vi "Beat.vi"(7 "Name (\"\" to Use UUID)":string="Beat") -> ()   [LabVIEW 2025]
doc: "Compact code template used to create a CSM module with a user interface. This template includes a user Event Structure for responding to user actions. The functionality of this template is identical to the CSM User Interface(UI) Module Template VI.\n\n\n> [!NOTE] <b>CSM Naming Rules</b>\n>\n> - CSM module name must be unique. Otherwise, CSM enters a `Critical Error` state.\n> - If the input module name is an empty string (\"\"), the system uses a UUID as the module name. Such a module is marked as standalone mode and does not appear in the module list.\n> - Worker Mode Rule: If the input module name ends with `#`, a worker mode node will be instantiated. Multiple worker mode nodes can form a worker mode module.\n> - Chain of Responsibility Mode Rule: If the input module name ends with `$` followed by a number, a chain of responsibility mode node will be instantiated. Multiple chain of responsibility mode nodes can form a chain of responsibility mode module.\n> - System-Level Module Rule: If the input module name starts with `.`, the module is a system-level module. Under default settings, such modules are not listed by the CSM - List Modules VI and are suitable for instantiating modules that run in the background.\n> - Submodule Rule: `.` is also allowed in a module name to separate the module name into multiple parts. CSM does not have strict rules for submodules. The `.` in the module name only marks the logical relationship between different modules. From an execution perspective, they are considered independent modules. The only difference is that you can obtain a list of logical submodules via the CSM - List Submodules VI.\n\n\n-- <b>Controls</b> --\n- <b>Name (\"\" to use UUID)</b>: CSM module name. Refer to <b>CSM Naming Rules</b> for module naming rules."
uses:
  <userlib>/_NEVSTOP/Communicable State Machine(CSM)/AdvanceAPI/CSM - Revert Arguments-Safe String.vi
  <userlib>/_NEVSTOP/Communicable State Machine(CSM)/_Shared/Trim Single-line Text.vi
  <userlib>/_NEVSTOP/Communicable State Machine(CSM)/AdvanceAPI/CSM - Break Down Multiple States String.vi
  <userlib>/_NEVSTOP/Communicable State Machine(CSM)/AdvanceAPI/CSM - Compact Multiple States.vi
  <userlib>/_NEVSTOP/Communicable State Machine(CSM)/AdvanceAPI/CSM - Make String Arguments Safe.vi
  <userlib>/_NEVSTOP/Communicable State Machine(CSM)/AdvanceAPI/CSM - Keywords.vi
  <userlib>/_NEVSTOP/Communicable State Machine(CSM)/Communicable State Machine.lvlib
panel:
  out "Next Beat":dbl
  out "Current Time":u32
  out "x >= y?":bool
  out "N":i32
  out "BeatInterval Indicator":dbl
  out "T0 indicator":dbl
  out "BeatActive":bool
  out "To exit":bool
  out "State History":string
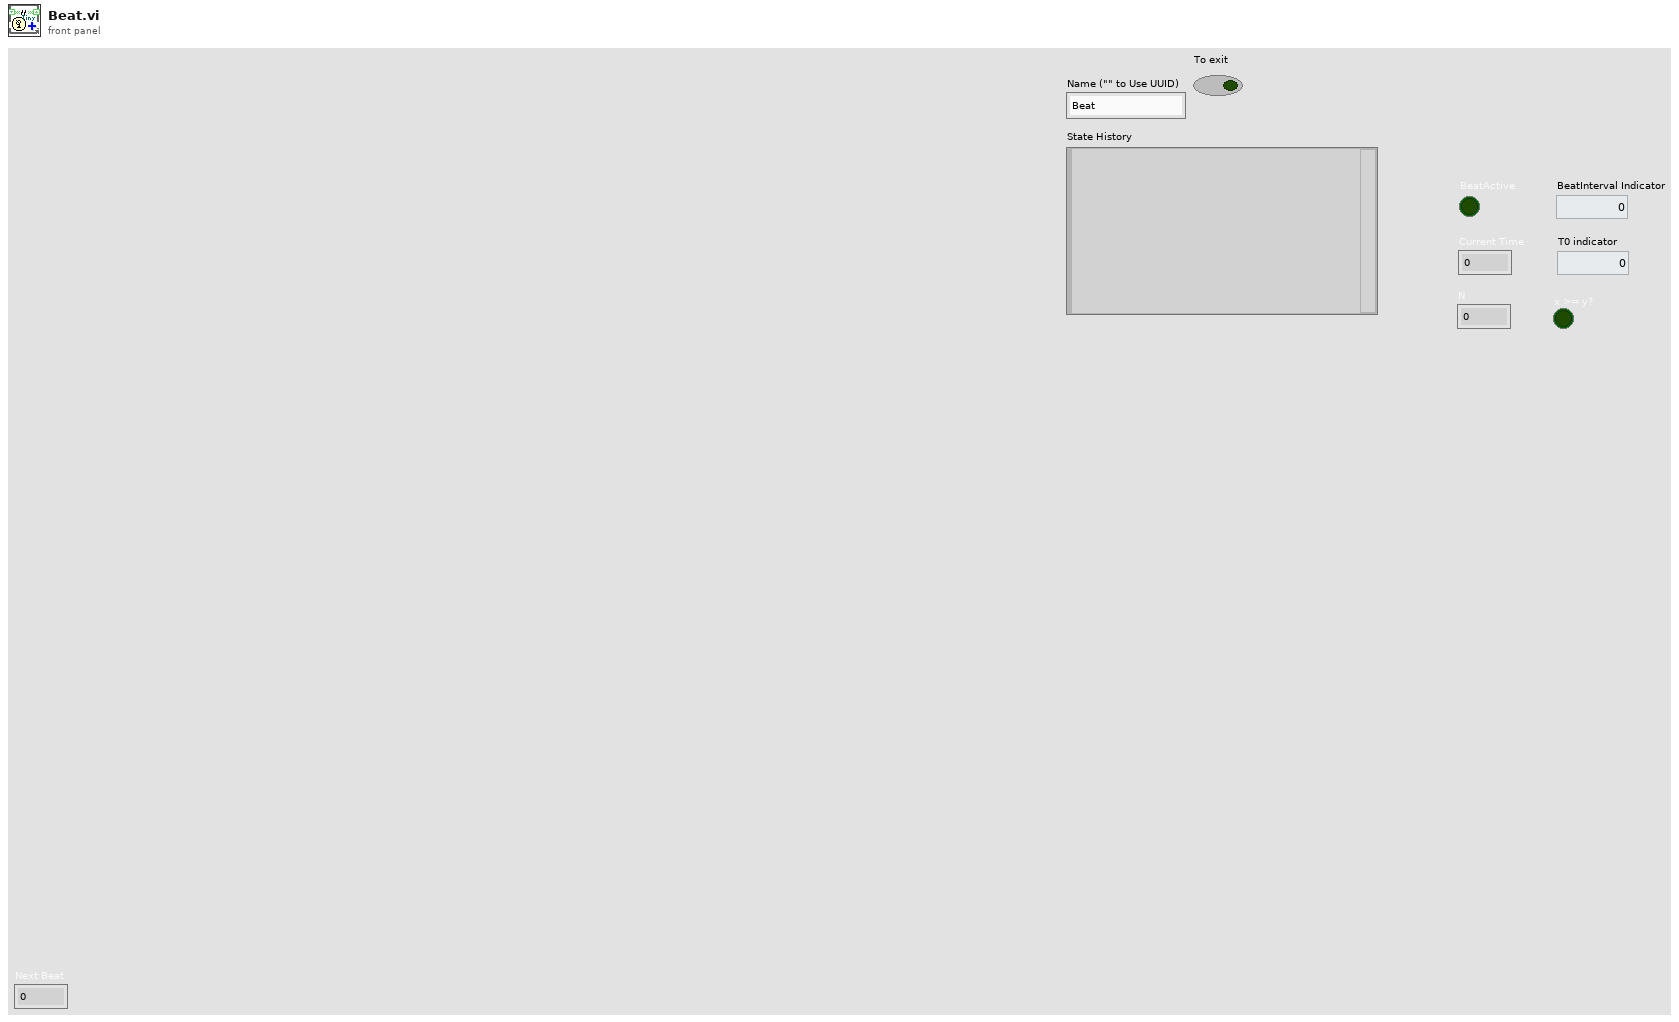
[diagram p1: front panel]
types:
  T1 = enum32{"Invalid", "Standard", "Closed", "Hidden", "Minimized", "Maximized"}
  T2 = enum32{"invalid app kind", "Development System", "Run Time System", "Student Edition", "Embedded LabVIEW", "Evaluation", "Custom"}
  T3 = typedef "Communicable State Machine.lvlib/_CSM_Response Source Message.ctl" = cluster{"‘State":string, "’Arguments":string, "’Error":errorcluster}
  T4 = cluster{"Current VI Reference":refnum<vi>, "Close Panel on Exit?":bool}
  T5 = cluster{"Core":cluster{"Current VI Reference":refnum<vi>, "Close Panel on Exit?":bool}, "T0":u32, "BeatInterval":i32, "BeatActive":bool}
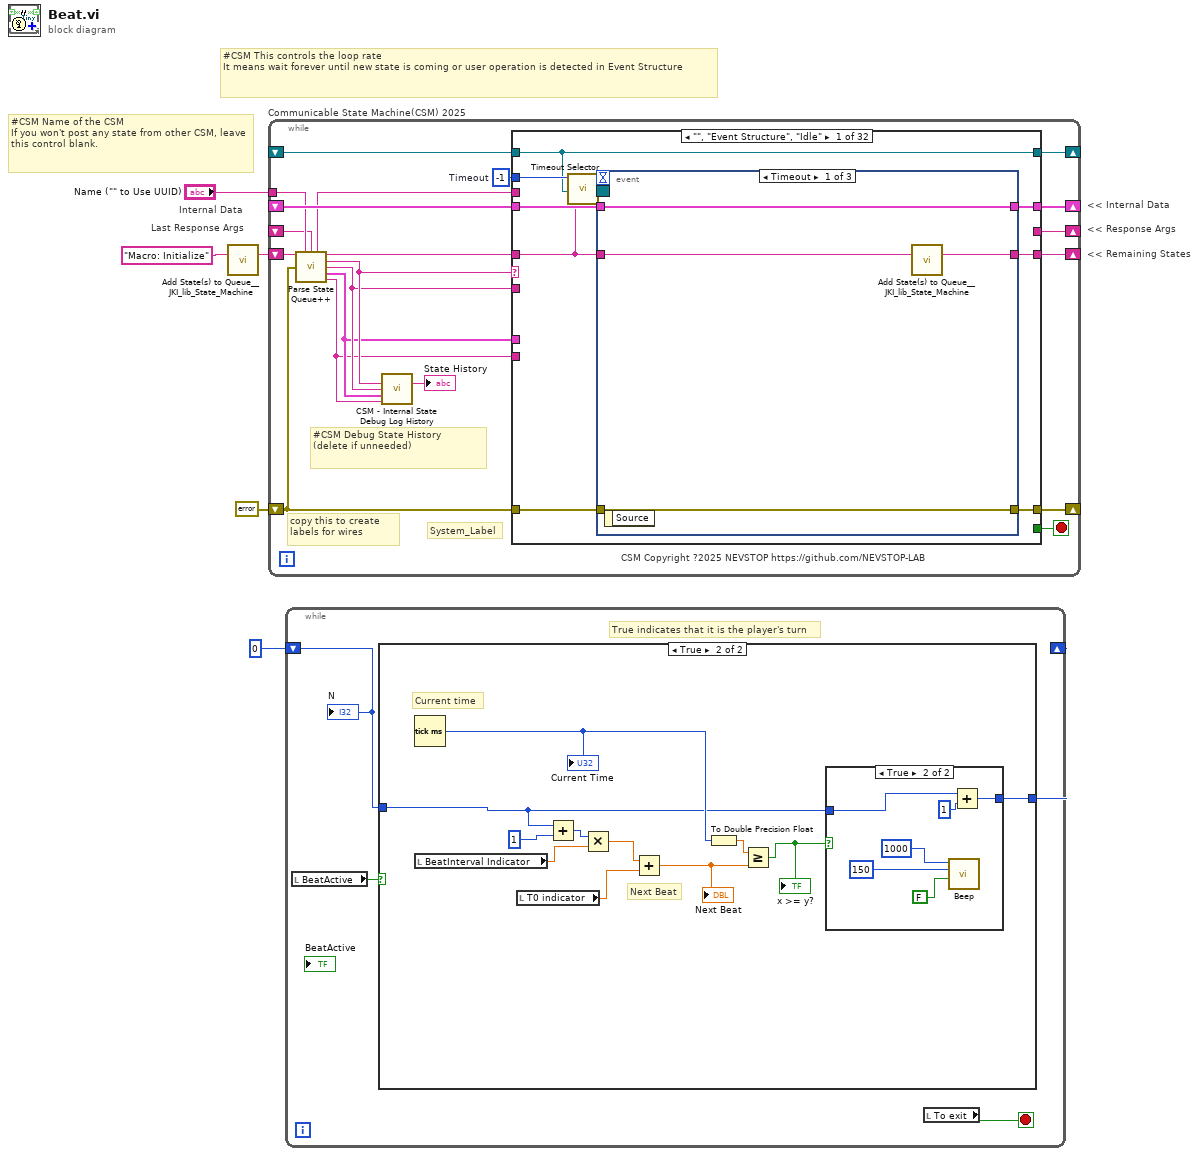
[diagram p0: block diagram]
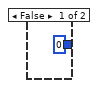
[diagram p2: hidden frame]
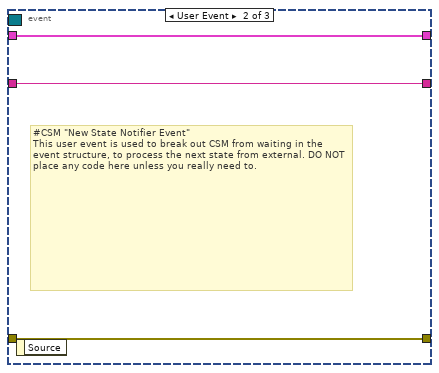
[diagram p4: hidden frame]
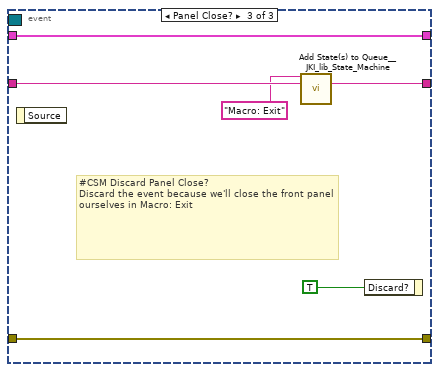
[diagram p5: hidden frame]
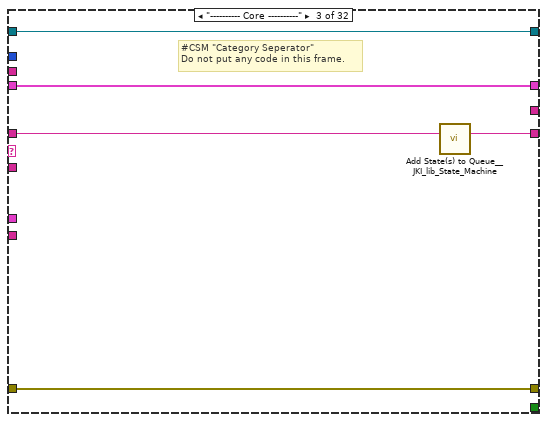
[diagram p7: hidden frame]
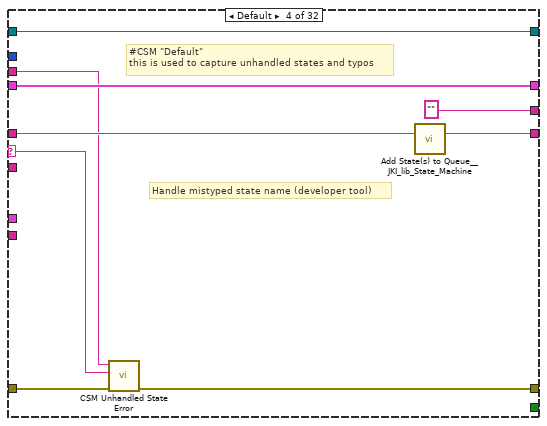
[diagram p8: hidden frame]
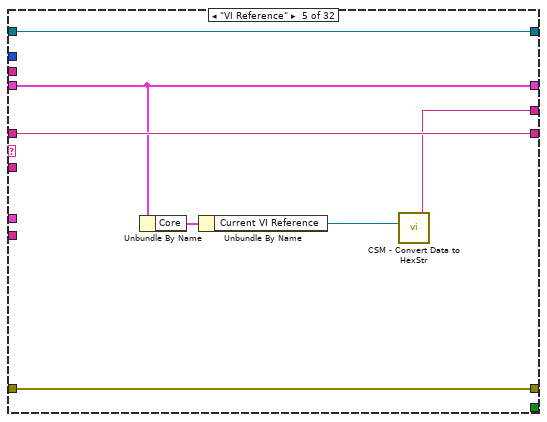
[diagram p9: hidden frame]
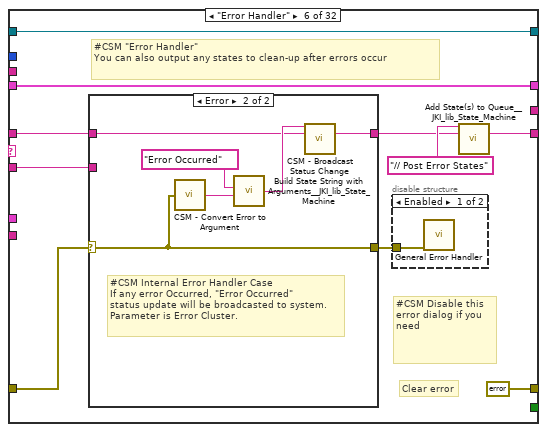
[diagram p10: hidden frame]
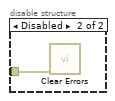
[diagram p11: hidden frame]
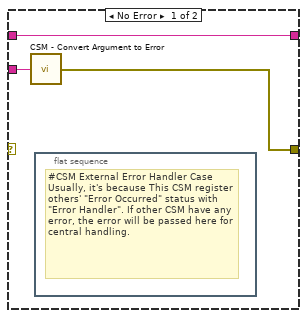
[diagram p12: hidden frame]
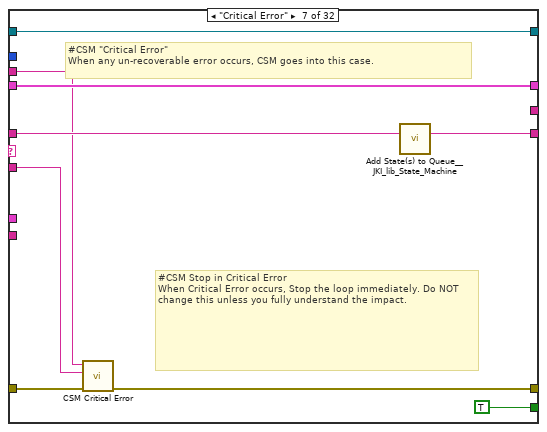
[diagram p13: hidden frame]
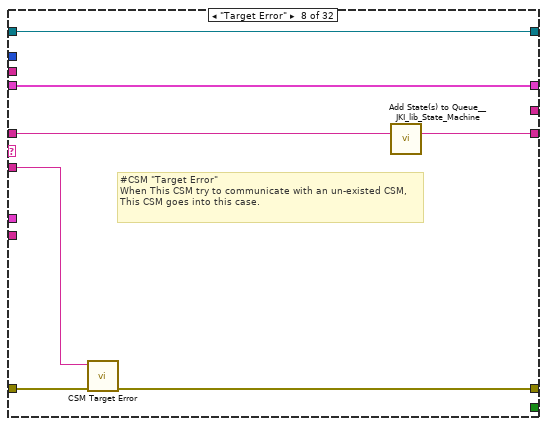
[diagram p14: hidden frame]
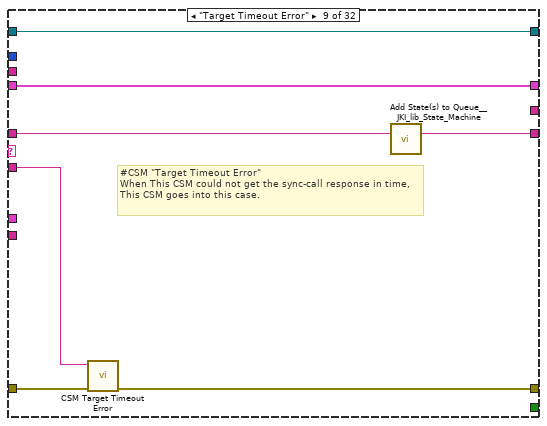
[diagram p15: hidden frame]
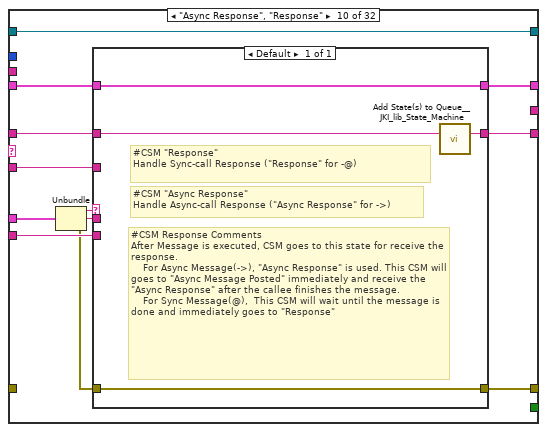
[diagram p16: hidden frame]
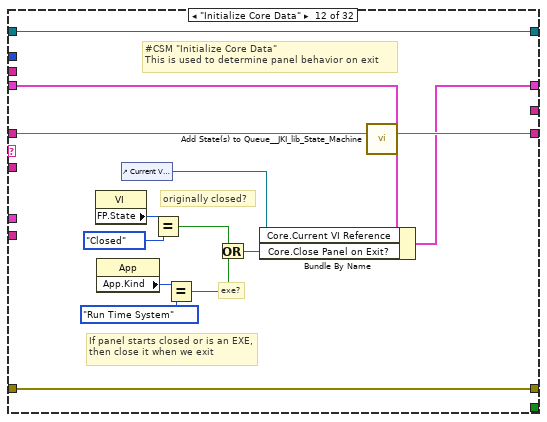
[diagram p18: hidden frame]
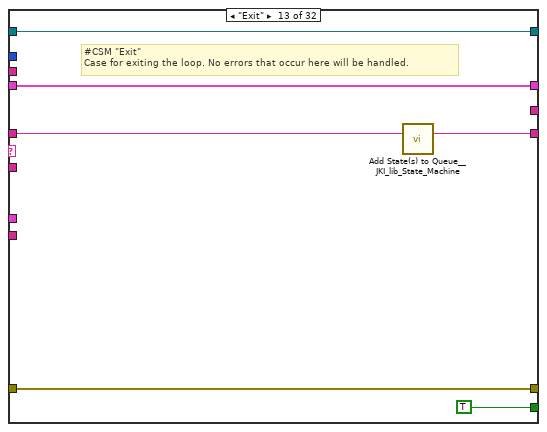
[diagram p19: hidden frame]
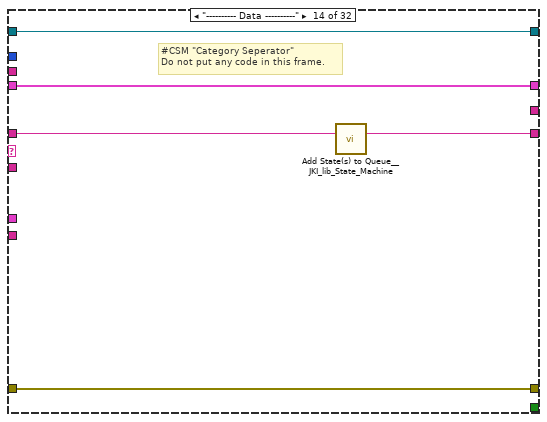
[diagram p20: hidden frame]
diagram:
  # "Last Response Args"
  # "Internal Data"
  # "#CSM Name of the CSM\nIf you won't post any state from other CSM, leave this control blank."
  # "#CSM This controls the loop rate\nIt means wait forever until new state is coming or user operation is detected in Event Structure"
  # "<< Internal Data"
  # "<< Response Args"
  # "<< Remaining States"
  n1 = call <vilib>:"Add State(s) to Queue__JKI_lib_State_Machine.vi"("State(s) in (\"\")"="Macro: Initialize" ("Init State(\"Macro: Initialize\")")) -> ("States Out"=w5:string)  [unwired: 14 in]
  n2 = while "Communicable State Machine(CSM) 2025" {
    shift-right: [w20] -> _
    shift-left: _ -> [w19]
    shift-right: [w23] -> _
    shift-left: errorcluster {"status"=FALSE, "code"=0, "source"=""} ("error out") -> [w17]
    shift-right: [w22] -> _
    shift-left: w5 -> [w24]
    tunnel: "Name (\"\" to Use UUID)" -> [w13]
    shift-right: [w16] -> _
    shift-left: _ -> [w7]
    shift-right: [w15] -> _
    shift-left: _ -> [w14]
    stop <- w21 stop-if-true
    w18 = -1  # Timeout
    # "#CSM Debug State History\n(delete if unneeded)"
    # "copy this to create labels for wires"
    # "System_Label"
    # "CSM Copyright ?2025 NEVSTOP https://github.com/NEVSTOP-LAB"
    n3 = call <userlib>:"Parse State Queue++.vi"("State Queue"=w24, "Name (\"\" to Use UUID)"=w13, "Response Arguments"=w7, "Previous Error"=w17) -> ("Name Used"=w8:string, "Remaining States"=w25:string, "Current State"=w12:string, "Arguments"=w11:string, "Additional Information"=w10:T3, "Source CSM"=w9:string)  [unwired: 6 in]
    n4 = call <userlib>:"CSM - Internal State Debug Log History.vi"("State"=w12, "Arguments (\"\")"=w11, ">> Response Source Message >>"=w10, "Source (\"\")"=w9) -> ("Debug Log"=→"State History":string)  [unwired: 11 in]
    n5 = case shown="\"\", \"Event Structure\", \"Idle\"" w12 {
      selector: w12 -> [_ _ _ w59 _ _ _ _ _ _ _ _ _ _ _ _ _ _ _ _ _ _ _ _ _ _ _ _ _ _ _ _]
      tunnel: w25 -> [w26 w50 w56 w64 w71 w77 w100 w106 w113 w122 w135 w150 w156 w161 w170 w177 w182 w189 w193 w199 w204 w211 w227 w297 w303 w315 w318 w334 w338 w349 w357 w362]
      tunnel: w11 -> [_ _ _ _ _ w76 w95 w105 w112 w121 _ _ _ _ _ _ _ _ _ _ _ w206 w221 _ _ _ _ w328 _ _ _ _]
      tunnel: w19 -> [w33 w49 w53 w62 w70 w81 w101 w108 w115 w124 w134 w143 w154 w158 _ w172 w179 w188 w192 w196 w202 w209 w223 w294 w300 w312 w317 w331 w343 w346 w353 w359]
      tunnel: [w32 w51 w54 w57 w72 errorcluster {"status"=FALSE, "code"=0, "source"=""} ("error out") w96 w103 w110 w127 w136 w147 w153 w159 w167 w173 w180 w183 w191 w197 w201 w207 w224 w295 w301 w313 w319 w335 w344 w347 w355 w360] -> w23
      tunnel: w17 -> [w31 w51 w54 w65 w72 w78 w102 w104 w111 _ w136 w147 w153 w159 w167 w174 w180 _ w194 w197 w201 w208 w225 w295 w301 w313 w319 w335 w344 w347 w355 w360]
      tunnel: [w34 w50 w55 w63 w71 w73 w99 w109 w116 w123 w135 w149 w155 w160 w169 w176 w181 w189 w193 w198 w203 w210 w226 w296 w302 w314 w318 w334 w337 w348 w356 w361] -> w22
      tunnel: [_ _ _ _ _ _ TRUE _ _ _ _ _ TRUE _ _ _ _ _ _ _ _ _ _ _ _ _ _ _ _ _ _ _] -> w21
      tunnel: [w30 w49 w53 w62 w70 w81 w101 w108 w115 w125 w134 w148 w154 w158 w168 w172 w179 w188 w192 w196 w202 w209 w223 w294 w300 w312 w317 w330 w343 w346 w350 w359] -> w20
      tunnel: w18 -> [w29 _ _ _ _ _ _ _ _ _ _ _ _ _ _ _ _ _ _ _ _ _ _ _ _ _ _ _ _ _ _ _]
      tunnel: w9 -> [_ _ _ _ _ _ _ _ _ w119 _ _ _ _ _ _ _ _ _ _ _ _ _ _ _ _ _ _ _ _ _ _]
      tunnel: w10 -> [_ _ _ _ _ _ _ _ _ w126 _ _ _ _ _ _ _ _ _ _ _ _ _ _ _ _ _ _ _ _ _ _]
      tunnel: [_ _ _ "" w66 _ _ _ _ _ _ _ _ _ _ _ _ _ _ _ _ _ _ _ _ _ _ "API1 Response" "API2 Response" _ _ _] -> w16
      tunnel: [w28 w48 w52 w60 w69 w80 w97 w107 w114 w128 w133 w137 w151 w157 w165 w171 w178 w187 w190 w195 w200 w205 w220 w293 w298 w305 w316 w333 w342 w345 w354 w358] -> w15
      tunnel: w14 -> [w28 w48 w52 w60 w69 w80 w97 w107 w114 w128 w133 w137 w151 w157 w165 w171 w178 _ w190 w195 w200 w205 w220 w293 w298 w305 w316 w333 w342 w345 w354 w358]
      tunnel: w8 -> [_ _ _ w58 _ _ w94 _ _ _ _ _ _ _ _ _ _ w186 _ _ _ _ _ _ _ _ _ _ _ _ _ _]
      frame "", "Event Structure", "Idle" {
        n6 = call <userlib>:"Timeout Selector.vi"("Remaining States"=w26, "Timeout Expected"=w29) -> ("Timeout"=w27:i32)  [unwired: 5 in]
        n7 = event shown="[0] Timeout" {
          selector: w28 -> [_ _ _]
          dyn-events: _ -> [_ _ _]
          timeout: w27 -> [_ _ _]
          tunnel: w26 -> [w38 w40 w47]
          tunnel: [w37 w40 w46] -> w34
          tunnel: w33 -> [w35 w41 w44]
          tunnel: [w36 w39 w45] -> w32
          tunnel: w31 -> [w36 w39 w45]
          tunnel: [w35 w41 w44] -> w30
          event Timeout {
            n8 = event-data() -> ()  [unwired: 1 in, 1 out]
            n9 = call <vilib>:"Add State(s) to Queue__JKI_lib_State_Machine.vi"("State(s) in (\"\")"=w38) -> ("States Out"=w37:string)  [unwired: 14 in]
          }
          event User Event {
            # "#CSM \"New State Notifier Event\"\nThis user event is used to break out CSM from waiting in the event structure, to process the next state from external. DO NOT place any code here unless you really need to."
            n10 = event-data() -> ()  [unwired: 1 in, 1 out]
          }
          event Panel Close? {
            # "#CSM Discard Panel Close?\nDiscard the event because we'll close the front panel ourselves in Macro: Exit"
            n11 = event-data() -> ()  [unwired: 1 in, 1 out]
            n12 = call <vilib>:"Add State(s) to Queue__JKI_lib_State_Machine.vi"("State(s) in Front (\"\")"="Macro: Exit", "State(s) in (\"\")"=w47) -> ("States Out"=w46:string)  [unwired: 13 in]
            n13 = event-data("Discard?"=TRUE) -> ()  [unwired: 1 in, 1 out]
          }
        }
      }
      frame "CSM Documentation" {
        # "#CSM README FIRST\n\nCommunicable State Machine(CSM) is a LabVIEW application framework that builds upon JKI State Machine(JKISM). It follows the pattern of JKISM and extends the keywords to describe message communication between modules, including concepts such as Sync-Message, Async-Message, Subscription/Unsubscription of status - essential elements for creating reusable code modules. For more information, please visit the CSM wiki: https://nevstop-lab.github.io/CSM-Wiki/\n\nFor instructions on JKI State Machine, visit: http://jki.net/state-machine/\nFor information about CSM, visit: https://github.com/NEVSTOP-LAB"
        # "#CSM \"Documentation\"\nCase for holding CSM Documenation"
      }
      frame "---------- Core ----------" {
        # "#CSM \"Category Seperator\"\nDo not put any code in this frame."
        n14 = call <vilib>:"Add State(s) to Queue__JKI_lib_State_Machine.vi"("State(s) in (\"\")"=w56) -> ("States Out"=w55:string)  [unwired: 14 in]
      }
      frame Default {
        # "#CSM \"Default\"\nthis is used to capture unhandled states and typos"
        # "Handle mistyped state name (developer tool)"
        n15 = call <userlib>:"CSM Unhandled State Error.vi"("error in (no error)"=w65, "Undefined State"=w59, "CSM Name"=w58) -> ("error out"=w57:errorcluster)  [unwired: 8 in]
        n16 = call <vilib>:"Add State(s) to Queue__JKI_lib_State_Machine.vi"("State(s) in (\"\")"=w64) -> ("States Out"=w63:string)  [unwired: 14 in]
      }
      frame "VI Reference" {
        n17 = Unbundle By Name(w70) -> ("Core"=w68:T4)
        n18 = Unbundle By Name(w68) -> ("Current VI Reference"=w67:refnum<vi>)
        n19 = call <userlib>:"CSM - Convert Data to HexStr.vi"("Variant"=w67) -> ("HEX String (0-9,A-F)"=w66:string)  [unwired: 8 in]
      }
      frame "Error Handler" {
        # "#CSM Disable this error dialog if you need"
        # "#CSM \"Error Handler\"\nYou can also output any states to clean-up after errors occur"
        # "Clear error"
        n20 = case shown="Error" w78 {
          selector: w78 -> [_ w88]
          tunnel: [w87 w90] -> w74
          tunnel: w77 -> [w87 w89]
          tunnel: w76 -> [w86 _]
          tunnel: [w85 w88] -> w79
          frame No Error {
            n21 = call <userlib>:"CSM - Convert Argument to Error.vi"("Argument"=w86) -> ("Error"=w85:errorcluster)  [unwired: 4 in]
            n22 = flat-sequence {
              frame #0 {
                # "#CSM External Error Handler Case\nUsually, it's because This CSM register others' \"Error Occurred\" status with \"Error Handler\". If other CSM have any error, the error will be passed here for central handling."
              }
            }
          }
          frame Error {
            # "#CSM Internal Error Handler Case \nIf any error Occurred, \"Error Occurred\" \nstatus update will be broadcasted to system.\nParameter is Error Cluster."
            n23 = call <userlib>:"CSM - Convert Error to Argument.vi"("Error"=w88) -> ("Argument"=w92:string)  [unwired: 4 in]
            n24 = call <vilib>:"Build State String with Arguments__JKI_lib_State_Machine.vi"("Arguments (\"\")"=w92, "State"="Error Occurred" ("Status with Arguments")) -> ("State with Arguments"=w91:string)  [unwired: 4 in]
            n25 = call <userlib>:"CSM - Broadcast Status Change.vi"("Status With Arguments"=w91, "State Queue"=w89) -> ("Remaining States"=w90:string)  [unwired: 13 in]
          }
        }
        n26 = disable-structure shown="Enabled" {
          disable-tunnel: w79 -> [w83 w84]
          frame Enabled {
            n27 = call <vilib>:"General Error Handler.vi"("error in (no error)"=w83) -> ()  [unwired: 10 in, 5 out]
          }
          frame Disabled {
            n28 = call <vilib>:"Clear Errors.vi"("error in (no error)"=w84) -> ()  [unwired: 5 in, 2 out]
          }
        }
        n29 = call <vilib>:"Add State(s) to Queue__JKI_lib_State_Machine.vi"("State(s) in Front (\"\")"="// Post Error States", "State(s) in (\"\")"=w74) -> ("States Out"=w73:string)  [unwired: 13 in]
      }
      frame "Critical Error" {
        # "#CSM Stop in Critical Error\nWhen Critical Error occurs, Stop the loop immediately. Do NOT change this unless you fully understand the impact."
        # "#CSM \"Critical Error\"\nWhen any un-recoverable error occurs, CSM goes into this case."
        n30 = call <userlib>:"CSM Critical Error.vi"("error in (no error)"=w102, "Arugments (As Reason)"=w95, "CSM Name"=w94) -> ("error out"=w96:errorcluster)  [unwired: 8 in]
        n31 = call <vilib>:"Add State(s) to Queue__JKI_lib_State_Machine.vi"("State(s) in (\"\")"=w100) -> ("States Out"=w99:string)  [unwired: 14 in]
      }
      frame "Target Error" {
        # "#CSM \"Target Error\"\nWhen This CSM try to communicate with an un-existed CSM, This CSM goes into this case."
        n32 = call <userlib>:"CSM Target Error.vi"("error in (no error)"=w104, "Arguments (As CSM Name)"=w105) -> ("error out"=w103:errorcluster)  [unwired: 9 in]
        n33 = call <vilib>:"Add State(s) to Queue__JKI_lib_State_Machine.vi"("State(s) in (\"\")"=w106) -> ("States Out"=w109:string)  [unwired: 14 in]
      }
      frame "Target Timeout Error" {
        # "#CSM \"Target Timeout Error\"\nWhen This CSM could not get the sync-call response in time, This CSM goes into this case."
        n34 = call <userlib>:"CSM Target Timeout Error.vi"("error in (no error)"=w111, "Arguments (As CSM Name)"=w112) -> ("error out"=w110:errorcluster)  [unwired: 9 in]
        n35 = call <vilib>:"Add State(s) to Queue__JKI_lib_State_Machine.vi"("State(s) in (\"\")"=w113) -> ("States Out"=w116:string)  [unwired: 14 in]
      }
      frame "Async Response", "Response" {
        n36 = Unbundle(w126) -> ("‘State"=w120:string, "’Arguments"=w118:string, "’Error"=w117:errorcluster)
        n37 = case shown="Default" w120 {
          tunnel: [w132] -> w127
          tunnel: w117 -> [w132]
          tunnel: [w131] -> w125
          tunnel: w124 -> [w131]
          tunnel: [w129] -> w123
          tunnel: w122 -> [w130]
          tunnel: w121 -> [_]
          tunnel: w119 -> [_]
          tunnel: w118 -> [_]
          frame Default {
            # "#CSM Response Comments\nAfter Message is executed, CSM goes to this state for receive the response.\n    For Async Message(->), \"Async Response\" is used. This CSM will goes to \"Async Message Posted\" immediately and receive the \"Async Response\" after the callee finishes the message.\n    For Sync Message(@),  This CSM will wait until the message is done and immediately goes to \"Response\""
            # "#CSM \"Async Response\"\nHandle Async-call Response (\"Async Response\" for ->)"
            # "#CSM \"Response\"\nHandle Sync-call Response (\"Response\" for -@)"
            n38 = call <vilib>:"Add State(s) to Queue__JKI_lib_State_Machine.vi"("State(s) in (\"\")"=w130) -> ("States Out"=w129:string)  [unwired: 14 in]
          }
        }
      }
      frame "Async Message Posted" {
        # "#CSM \"Async Message Posted\"\nAfter Async Message is posted (-> or ->| ), CSM goes to this state for post-action.\nYou can use Argument - State to tell which Async Message is called."
      }
      frame "Initialize Core Data" {
        # "#CSM \"Initialize Core Data\"\nThis is used to determine panel behavior on exit"
        # "originally closed?"
        # "exe?"
        # "If panel starts closed or is an EXE, then close it when we exit"
        n39 = property class="VI"() -> ("FP.State"=w140:T1)  [unwired: 2 in, 2 out]
        n40 = property class="App"() -> ("App.Kind"=w146:T2)  [unwired: 2 in, 2 out]
        n41 = control-ref of="Current VI Reference"() -> (w141:refnum<vi>)
        n42 = Equal?(x=w140, y=T1."Closed" ("Front Panel Window:State")) -> (x = y?=w138:bool)
        n43 = Equal?(x=w146, y=T2."Run Time System" ("Application:Kind")) -> (x = y?=w144:bool)
        n44 = Or(x=w138, y=w144) -> (x .or. y?=w142:bool)
        n45 = Bundle By Name(cluster=w143, "Core.Current VI Reference"=w141, "Core.Close Panel on Exit?"=w142) -> (w148:T5)
        n46 = call <vilib>:"Add State(s) to Queue__JKI_lib_State_Machine.vi"("State(s) in (\"\")"=w150) -> ("States Out"=w149:string)  [unwired: 14 in]
      }
      frame "Exit" {
        # "#CSM \"Exit\"\nCase for exiting the loop. No errors that occur here will be handled."
        n47 = call <vilib>:"Add State(s) to Queue__JKI_lib_State_Machine.vi"("State(s) in (\"\")"=w156) -> ("States Out"=w155:string)  [unwired: 14 in]
      }
      frame "---------- Data ----------" {
        # "#CSM \"Category Seperator\"\nDo not put any code in this frame."
        n48 = call <vilib>:"Add State(s) to Queue__JKI_lib_State_Machine.vi"("State(s) in (\"\")"=w161) -> ("States Out"=w160:string)  [unwired: 14 in]
      }
      frame "Data: Initialize" {
        w162 = FALSE  # BeatActive
        w163 = 0  # BeatInterval
        w164 = u32 0  # T0
        w166 = T4 {"Current VI Reference"=refnum, "Close Panel on Exit?"=FALSE}  # Core
        # "#CSM do not delete - used by framework"
        # "#CSM Expand Bundle to add new data elements to shift register data."
        # "#CSM Add new data here."
        # "Initialize the shift-register data, here.\n(data names are defined by what you wire into the bundle function)"
        n49 = Bundle("Core"=w166, "T0"=w164, "BeatInterval"=w163, "BeatActive"=w162) -> (w168:T5)  [unwired: 1 in]
        n50 = call <vilib>:"Add State(s) to Queue__JKI_lib_State_Machine.vi"("State(s) in (\"\")"=w170) -> ("States Out"=w169:string)  [unwired: 14 in]
      }
      frame "Data: Cleanup" {
        # "Cleanup any data and references, here.\n(this is called automatically, by the Macro: Exit)"
        n51 = Unbundle By Name(w172) -> ("Core.Current VI Reference"=w175:refnum<vi>)
        n52 = Close Reference(reference=w175, error in (no error)=w174) -> (error out=w173:errorcluster)
        n53 = call <vilib>:"Add State(s) to Queue__JKI_lib_State_Machine.vi"("State(s) in (\"\")"=w177) -> ("States Out"=w176:string)  [unwired: 14 in]
      }
      frame "---------- Events ----------" {
        # "#CSM \"Category Seperator\"\nDo not put any code in this frame."
        n54 = call <vilib>:"Add State(s) to Queue__JKI_lib_State_Machine.vi"("State(s) in (\"\")"=w182) -> ("States Out"=w181:string)  [unwired: 14 in]
      }
      frame "Events: Register" {
        # "#CSM \"Events: Register\"\nRegister user event. New Message Event is registered to break CSM waiting in event structure by default."
        # "#CSM Register New Message Event\nRegister message event to break Waiting in Event structure."
        n55 = call <userlib>:"CSM - Get New State Notifier Event.vi"("Name (\"\" to Use UUID)"=w186) -> ("error out"=w184:errorcluster, "New State Notifier Event"=w185:refnum<user-event>)  [unwired: 9 in]
        n56 = register-events(error in=w184, w185) -> (reference out=w187:refnum<event-registration>, error out=w183:errorcluster)  [unwired: 1 in]
      }
      frame "Events: Unregister" {
        # "#CSM \"Events: Unregister\"\nUnregister user event."
        n57 = Unregister For Events(event registration refnum=w190, error in=w194) -> (error out=w191:errorcluster)
      }
      frame "---------- UI ----------" {
        # "#CSM \"Category Seperator\"\nDo not put any code in this frame."
        n58 = call <vilib>:"Add State(s) to Queue__JKI_lib_State_Machine.vi"("State(s) in (\"\")"=w199) -> ("States Out"=w198:string)  [unwired: 14 in]
      }
      frame "UI: Initialize" {
        # "#CSM \"UI: Initialize\"\nInitialize the User Interface, here.\n(this is called automatically, by the Macro: Init)"
        n59 = call <vilib>:"Add State(s) to Queue__JKI_lib_State_Machine.vi"("State(s) in (\"\")"=w204) -> ("States Out"=w203:string)  [unwired: 14 in]
      }
      frame "UI: Cursor Set" {
        # "#CSM \"UI: Cursor Set\"\nSet and Unset Cursor Busy.\n(Usage: \"UI: Cursor Set >> Busy|Idle\")"
        # "Argument"
        n60 = disable-structure shown="Default" {
          disable-tunnel: w208 -> [w214 w219]
          disable-tunnel: [w213 w219] -> w207
          disable-tunnel: w206 -> [w212 _]
          frame condition #0 (active) {
            n61 = case shown="\"Idle\", Default" w212 {
              tunnel: w214 -> [w216 w218]
              tunnel: [w215 w217] -> w213
              frame "Idle", Default {
                n62 = call <vilib>:"Unset Busy.vi"("error in (no error)"=w216) -> ("error out"=w215:errorcluster)  [unwired: 10 in]
              }
              frame "Busy" {
                n63 = call <vilib>:"Set Busy.vi"("error in (no error)"=w218) -> ("error out"=w217:errorcluster)  [unwired: 9 in, 1 out]
              }
            }
          }
          frame condition #1 {
          }
        }
        n64 = call <vilib>:"Add State(s) to Queue__JKI_lib_State_Machine.vi"("State(s) in (\"\")"=w211) -> ("States Out"=w210:string)  [unwired: 14 in]
      }
      frame "UI: Front Panel State" {
        # "#CSM \"UI: Front Panel State\"\nSet Front Panel Open or Closed\n(Usage: \"UI: Front Panel State >> Open|Close\")"
        # "Argument"
        n65 = Unbundle By Name(w223) -> ("Core.Current VI Reference"=w222:refnum<vi>)
        n66 = call <vilib>:"Add State(s) to Queue__JKI_lib_State_Machine.vi"("State(s) in (\"\")"=w227) -> ("States Out"=w226:string)  [unwired: 14 in]
        n67 = case shown="\"Close\", \"Closed\"" w221 {
          tunnel: w225 -> [w233 w248 w259 w272 w285]
          tunnel: [w235 w249 w261 w274 w287] -> w224
          tunnel: w222 -> [w234 w246 w260 w273 w286]
          frame "Open", "Standard", Default {
            w228 = T1."Standard" ("State")
            n68 = property class="VI"(reference=w234, error in=w233) -> (reference out=w231:refnum<vi>, error out=w232:errorcluster, "FP.State"=w230:T1)
            n69 = Not Equal?(x=w230, y=w228) -> (x != y?=w229:bool)
            n70 = case shown="True" w229 {
              tunnel: [w239 w241] -> w235
              tunnel: w232 -> [w238 w241]
              tunnel: w231 -> [w237 _]
              tunnel: w228 -> [w236 _]
              frame True {
                n71 = invoke class="VI" method="FP.Open"(reference=w237, error in=w238, "Activate"=TRUE, "State"=w236) -> (error out=w239:errorcluster)  [unwired: 1 in, 4 out]
              }
              frame False {
              }
            }
          }
          frame "Close", "Closed" {
            n72 = property class="VI"(reference=w246, error in=w248) -> (reference out=w245:refnum<vi>, error out=w247:errorcluster, "FP.State"=w243:T1)
            n73 = Not Equal?(x=w243, y=T1."Closed" ("Front Panel Window:State")) -> (x != y?=w242:bool)
            n74 = case shown="False" w242 {
              tunnel: [w250 w253] -> w249
              tunnel: w247 -> [w250 w252]
              tunnel: w245 -> [_ w251]
              frame False {
              }
              frame True {
                n75 = invoke class="VI" method="FP.Close"(reference=w251, error in=w252) -> (error out=w253:errorcluster)  [unwired: 1 in, 2 out]
              }
            }
          }
          frame "Hidden", "Hide" {
            w254 = T1."Hidden" ("State")
            n76 = property class="VI"(reference=w260, error in=w259) -> (reference out=w257:refnum<vi>, error out=w258:errorcluster, "FP.State"=w256:T1)
            n77 = Not Equal?(x=w256, y=w254) -> (x != y?=w255:bool)
            n78 = case shown="True" w255 {
              tunnel: [w265 w266] -> w261
              tunnel: w258 -> [w264 w266]
              tunnel: w257 -> [w263 _]
              tunnel: w254 -> [w262 _]
              frame True {
                n79 = invoke class="VI" method="FP.Open"(reference=w263, error in=w264, "State"=w262) -> (error out=w265:errorcluster)  [unwired: 2 in, 4 out]
              }
              frame False {
              }
            }
          }
          frame "Minimize", "Minimized" {
            w267 = T1."Minimized" ("State")
            n80 = property class="VI"(reference=w273, error in=w272) -> (reference out=w270:refnum<vi>, error out=w271:errorcluster, "FP.State"=w269:T1)
            n81 = Not Equal?(x=w269, y=w267) -> (x != y?=w268:bool)
            n82 = case shown="True" w268 {
              tunnel: [w278 w279] -> w274
              tunnel: w271 -> [w277 w279]
              tunnel: w270 -> [w276 _]
              tunnel: w267 -> [w275 _]
              frame True {
                n83 = invoke class="VI" method="FP.Open"(reference=w276, error in=w277, "State"=w275) -> (error out=w278:errorcluster)  [unwired: 2 in, 4 out]
              }
              frame False {
              }
            }
          }
          frame "Maximize", "Maximized" {
            w280 = T1."Maximized" ("State")
            n84 = property class="VI"(reference=w286, error in=w285) -> (reference out=w283:refnum<vi>, error out=w284:errorcluster, "FP.State"=w282:T1)
            n85 = Not Equal?(x=w282, y=w280) -> (x != y?=w281:bool)
            n86 = case shown="True" w281 {
              tunnel: [w291 w292] -> w287
              tunnel: w284 -> [w290 w292]
              tunnel: w283 -> [w289 _]
              tunnel: w280 -> [w288 _]
              frame True {
                n87 = invoke class="VI" method="FP.Open"(reference=w289, error in=w290, "State"=w288) -> (error out=w291:errorcluster)  [unwired: 2 in, 4 out]
              }
              frame False {
              }
            }
          }
        }
      }
      frame "---------- Macro ----------" {
        # "#CSM \"Category Seperator\"\nDo not put any code in this frame."
        n88 = call <vilib>:"Add State(s) to Queue__JKI_lib_State_Machine.vi"("State(s) in (\"\")"=w297) -> ("States Out"=w296:string)  [unwired: 14 in]
      }
      frame "Macro: Initialize" {
        w299 = "Data: Initialize\nInitialize Core Data\nEvents: Register\nUI: Initialize\nUI: Front Panel State >> Open\nAction: Hide Beat"  # Data: Initialize Initialize Core Data Events: Register UI: Initialize UI: Front Panel State >> Open Action: Hide Beat
        # "#CSM \"Macro: Initialize\"\nInitialization Macro (This is called once, when the VI starts)"
        n89 = call <vilib>:"Add State(s) to Queue__JKI_lib_State_Machine.vi"("State(s) in Front (\"\")"=w299, "State(s) in (\"\")"=w303) -> ("States Out"=w302:string)  [unwired: 13 in]
      }
      frame "Macro: Exit" {
        # "#CSM \"Macro: Exit\"\nExit Macro (This is called once, when the VI exits)"
        n90 = Unbundle By Name(w312) -> ("Core.Close Panel on Exit?"=w311:bool)
        n91 = Select(t="UI: Front Panel State >> Close", s=w311, f="") -> (s? t:f=w308:string)
        n92 = call <vilib>:"Add State(s) to Queue__JKI_lib_State_Machine.vi"("State(s) in Front (\"\")"="//Exit Sub-Modules ", "State(s) in (\"\")"=w308, "State(s) at Back (\"\")"="Data: Cleanup\nEvents: Unregister\nExit") -> ("States Out"=w306:string)  [unwired: 12 in]
        n93 = call <vilib>:"Add State(s) to Queue__JKI_lib_State_Machine.vi"("State(s) in Front (\"\")"=w306, "State(s) in (\"\")"=w315) -> ("States Out"=w314:string)  [unwired: 13 in]
      }
      frame "---------- API ----------" {
        # "#CSM \"Category Seperator\"\nDo not put any code in this frame."
      }
      frame "API: StartBeat" {
        # "Get T0 and BeatInterval\nfrom Game module"
        # "#CSM API Example\nCopy/Rename this case for your own API"
        # "#CSM Response\nConnect this to return the response of your API"
        # "#CSM >> Source CSM >>\nIf you need to tell who triggered this state , use this string. If it's this case itself, this string is \"\"."
        # "#CSM >> Arguments >>\nDeal with the parameter if any"
        n94 = Spreadsheet String To Array(delimiter (Tab)=",", format string="%d,%d", spreadsheet string=w328, array type (2D Dbl)=i32[] []) -> (array=w325:i32[])
        n95 = Index Array(array=w325, index #1=0 ("index"), index #2=1 ("index")) -> (element #1=w320:i32, element #2=w321:i32)
        "BeatInterval Indicator" <- w321
        "T0 indicator" <- w320
        n96 = Bundle By Name(cluster=w331, "T0"=w320, "BeatInterval"=w321) -> (w330:T5)
        n97 = local write "BeatActive"(TRUE) -> ()
      }
      frame "API: StopBeat" {
        # "#CSM API Example\nCopy/Rename this case for your own API"
        # "unpack Hex String  to Variant\nif complex parameter is needed."
        n98 = local write "BeatActive"(FALSE) -> ()
        n99 = call <vilib>:"Add State(s) to Queue__JKI_lib_State_Machine.vi"("State(s) in Front (\"\")"="Macro: Exit" ("State(s) in Front (\"\")"), "State(s) in (\"\")"=w338) -> ("States Out"=w337:string)  [unwired: 13 in]
        "To exit" <- TRUE
      }
      frame "---------- Action ----------" {
        # "#CSM \"Category Seperator\"\nDo not put any code in this frame."
        n100 = call <vilib>:"Add State(s) to Queue__JKI_lib_State_Machine.vi"("State(s) in (\"\")"=w349) -> ("States Out"=w348:string)  [unwired: 14 in]
      }
      frame "Action: Hide Beat" {
        # "#CSM \"Internal State\"\nThis category is used for holding internal states"
        n101 = property class="VI"("FP.State"=T1."Hidden" ("Front Panel Window:State")) -> (reference out=w352:refnum<vi>)  [unwired: 2 in, 1 out]
        n102 = Bundle By Name(cluster=w353, "Core.Current VI Reference"=w352) -> (w350:T5)
        n103 = call <vilib>:"Add State(s) to Queue__JKI_lib_State_Machine.vi"("State(s) in (\"\")"=w357) -> ("States Out"=w356:string)  [unwired: 14 in]
      }
      frame "Action: action2" {
        # "#CSM \"Internal State\"\nThis category is used for holding internal states"
        n104 = call <vilib>:"Add State(s) to Queue__JKI_lib_State_Machine.vi"("State(s) in (\"\")"=w362) -> ("States Out"=w361:string)  [unwired: 14 in]
      }
    }
  }
  n105 = while {
    shift-right: [w364] -> _
    shift-left: 0 -> [w365]
    stop <- w363 stop-if-true
    # "True indicates that it is the player's turn"
    n106 = local read "BeatActive"() -> (w366:bool)
    n107 = case shown="True" w366 {
      tunnel: w365 -> [_ w370]
      tunnel: [0 w374] -> w364
      frame False {
      }
      frame True {
        # "Next Beat"
        # "Current time"
        n108 = Tick Count (ms)() -> (millisecond timer value=w372:u32)
        "Current Time" <- w372
        n109 = local read "BeatInterval Indicator"() -> (w378:dbl)
        n110 = local read "T0 indicator"() -> (w376:dbl)
        n111 = Add(x=w370, y=1) -> (x+y=w368:i32)
        n112 = Multiply(x=w368, y=w378) -> (x*y=w377:dbl)
        n113 = Add(x=w377, y=w376) -> (x+y=w373:dbl)
        "Next Beat" <- w373
        n114 = To Double Precision Float(number=w372) -> (double precision float=w371:dbl)
        n115 = Greater Or Equal?(x=w371, y=w373) -> (x >= y?=w375:bool)
        "x >= y?" <- w375
        n116 = case shown="True" w375 {
          tunnel: w370 -> [w379 w383]
          tunnel: [w379 w381] -> w374
          frame False {
          }
          frame True {
            n117 = call <vilib>:"Beep.vi"("use system alert? (T)"=FALSE, "duration (msec)"=u32 150, "frequency (Hz)"=u32 1000) -> ()  [unwired: 9 in]
            n118 = Add(x=w383, y=1) -> (x+y=w381:i32)
          }
        }
      }
    }
    n119 = local read "To exit"() -> (w363:bool)
    "N" <- w365
  }
